vi "Instrument Face Avant.vi"() -> ()   [LabVIEW 2024]
uses:
  <instrlib>/Keithley 2000/Keithley 2000.lvlib
panel:
  in  "Bouton Arrêt du processus":bool
  out "Valeur moyenne":dbl
  out "Valeur max":dbl
  out "Valeur min":dbl
  out "Chaîne":string
  out "Fichier de mesure":path
  out "Graphe":dbl[](graph)
  in  "Nombre de mesures ?":dbl=1.0 min=1.0 step=1.0
  in  "Période (s) ?":dbl=1.0 min=1.0 step=1.0
  in  "Bouton EXECUTER":bool
  in  "Bouton CONFIGURER":bool
  in  "Fonction":u16(ring) items=["TENSION DC", "TENSION AC", "COURANT DC", "COURANT AC", "RESISTANCE 2 points", "RESISTANCE 4 points", "FREQUENCE", "TEMPERATURE"]
  in  "Message d'accueil":string(combo)
  # "MODULE D'ACQUISITION ET DE TRAITEMENT DE DONNEES"
  # "RESULTATS DES MESURES"
  # "CONFIGURATION DE L'INSTRUMENT"
  # "CONFIGURATION DE L'ACQUISITION"
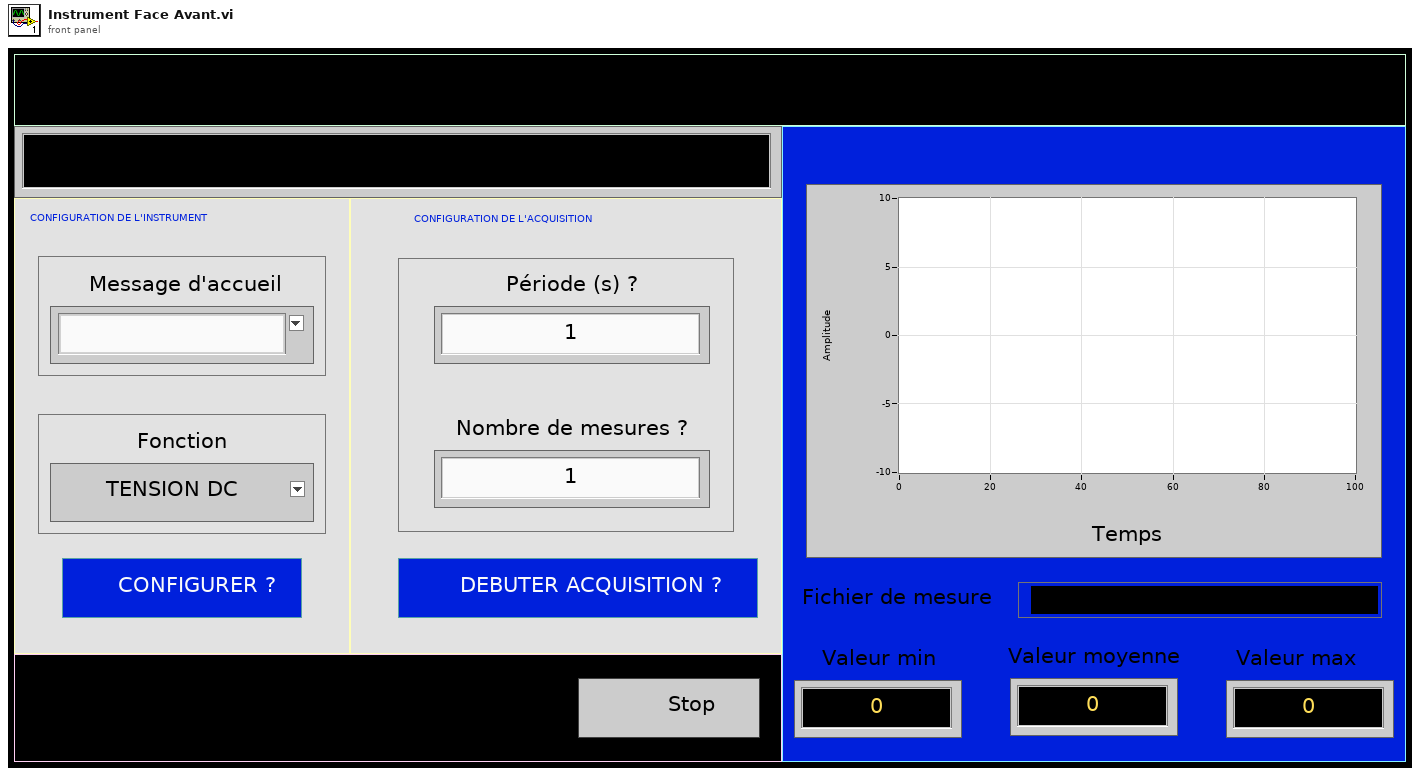
[diagram p1: front panel]
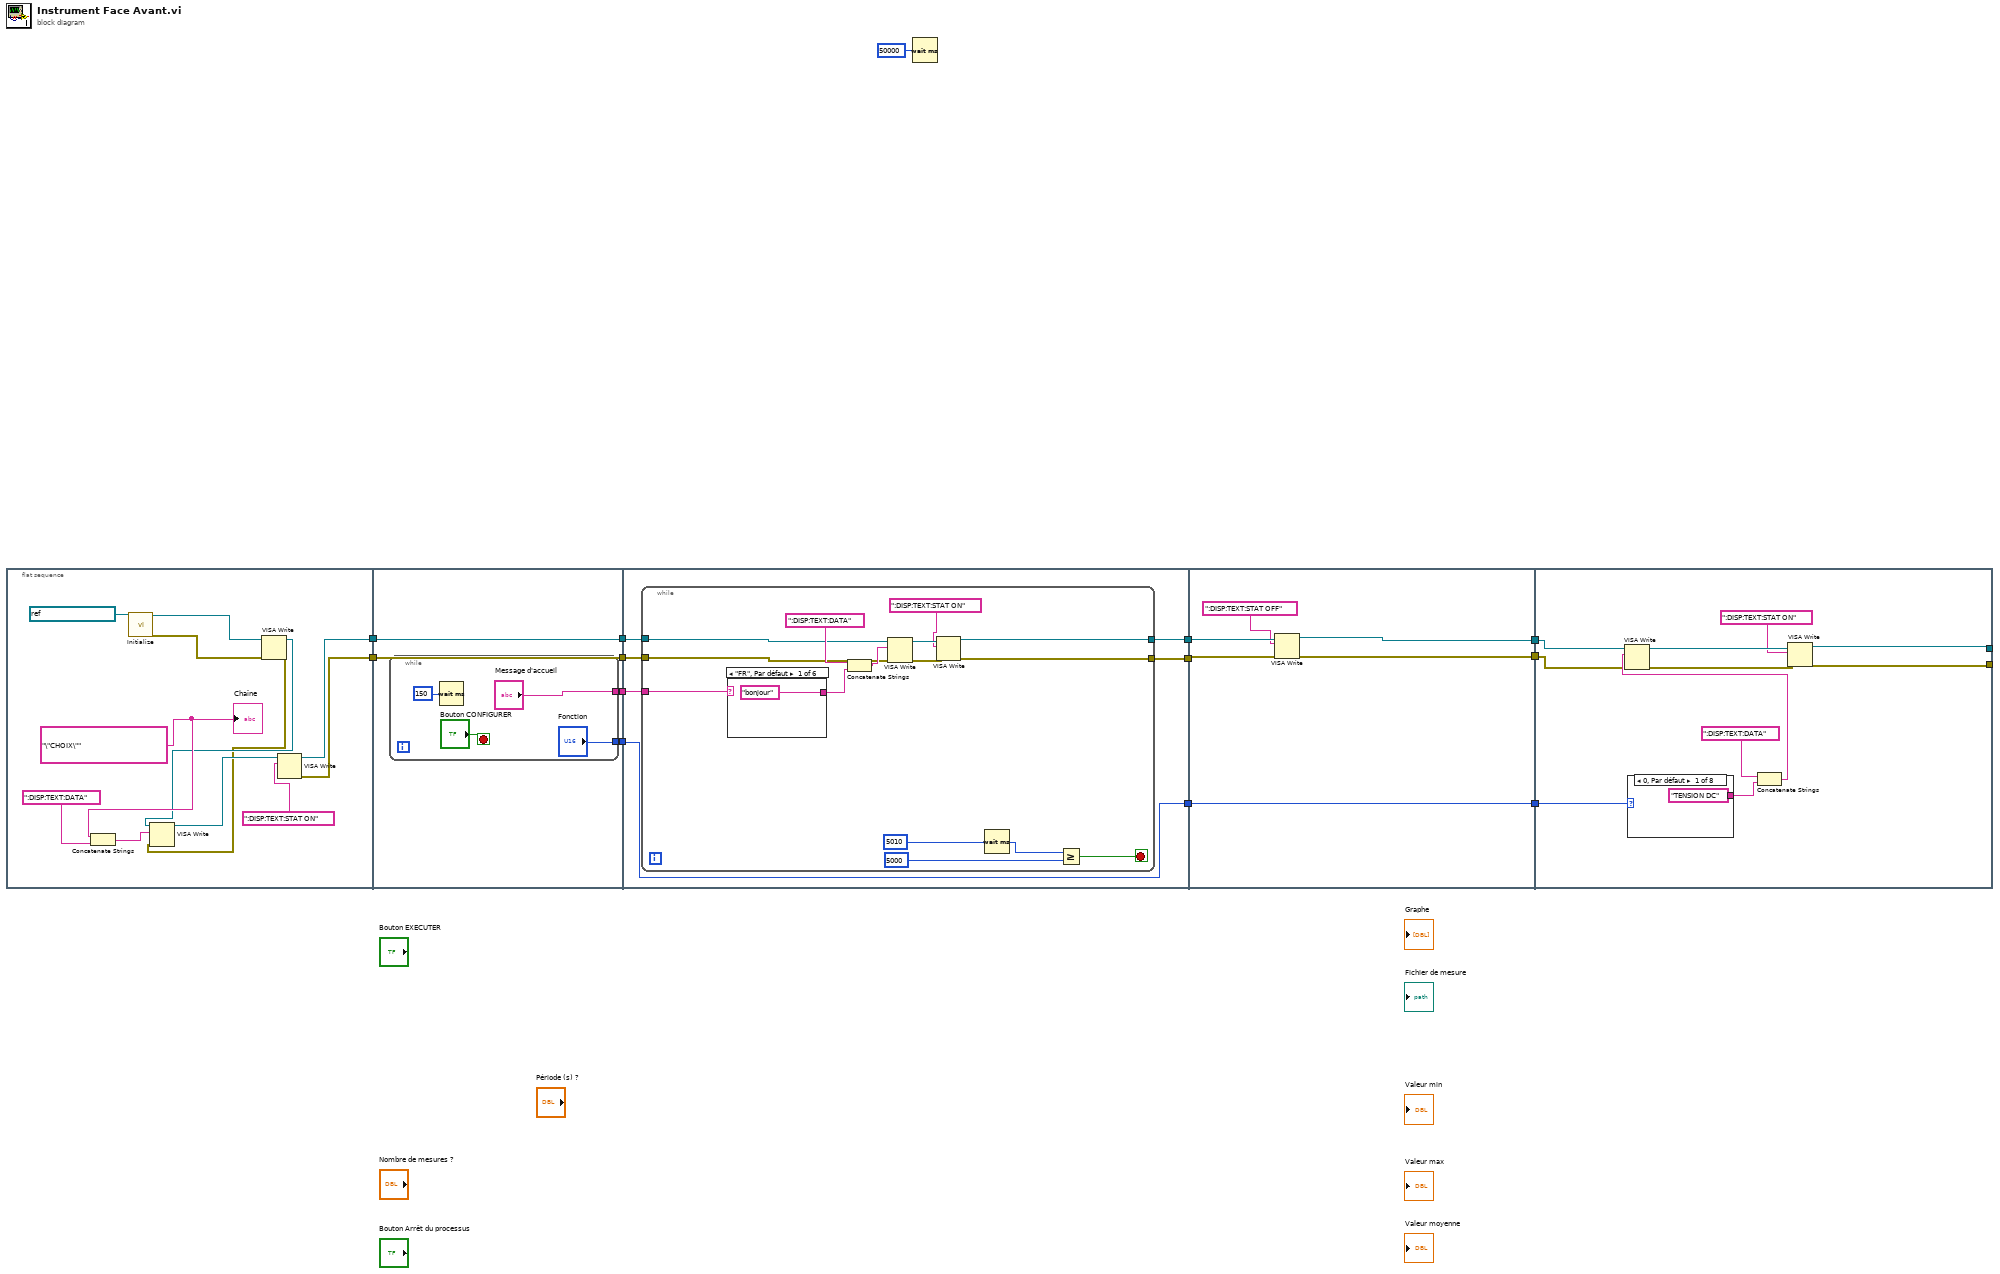
[diagram p0: block diagram]
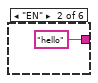
[diagram p2: hidden frame]
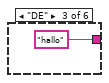
[diagram p3: hidden frame]
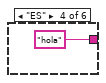
[diagram p4: hidden frame]
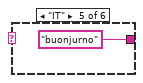
[diagram p5: hidden frame]
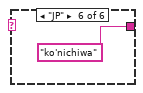
[diagram p6: hidden frame]
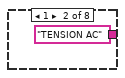
[diagram p7: hidden frame]
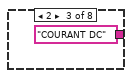
[diagram p8: hidden frame]
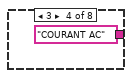
[diagram p9: hidden frame]
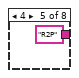
[diagram p10: hidden frame]
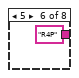
[diagram p11: hidden frame]
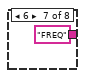
[diagram p12: hidden frame]
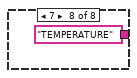
[diagram p13: hidden frame]
diagram:
  n1 = flat-sequence {
    tunnel: [w16] -> w12
    tunnel: [w17] -> w10
    tunnel: [w29] -> w13
    tunnel: w12 -> [w29]
    tunnel: [w28] -> w11
    tunnel: w10 -> [w28]
    tunnel: [w27] -> w5
    tunnel: [w26] -> w2
    tunnel: w13 -> [w39]
    tunnel: w11 -> [w38]
    tunnel: [w37] -> w9
    tunnel: [w36] -> w8
    tunnel: w5 -> [w35]
    tunnel: [w34] -> w3
    tunnel: w2 -> [w34]
    tunnel: w9 -> [w64]
    tunnel: w8 -> [w66]
    tunnel: [w65] -> w7
    tunnel: [w63] -> w6
    tunnel: [w61] -> w4
    tunnel: w3 -> [w61]
    tunnel: w7 -> [w74]
    tunnel: w6 -> [w73]
    tunnel: [w69] -> _
    tunnel: [w68] -> _
    tunnel: w4 -> [w67]
    frame #0 {
      w20 = "\"CHOIX\""
      n2 = Concatenate Strings(w20, ":DISP:TEXT:DATA" ("chaîne")) -> (w22:string)
      n3 = call <instrlib>:"Initialize.vi"("VISA resource name"=refnum<visa-resource-name> "GPIB0::2::INSTR") -> ("VISA resource name out"=w24:refnum<visa-resource-name>, "error out"=w23:errorcluster)  [unwired: 17 in]
      n4 = VISA Write(VISA resource name=w24, error in (no error)=w23) -> (VISA resource name out=w15:refnum<visa-resource-name>, error out=w14:errorcluster)  [unwired: 1 in, 1 out]
      n5 = VISA Write(VISA resource name=w15, write buffer=w22, error in (no error)=w14) -> (VISA resource name out=w19:refnum<visa-resource-name>)  [unwired: 2 out]
      n6 = VISA Write(VISA resource name=w19, write buffer=":DISP:TEXT:STAT ON" ("chaîne")) -> (VISA resource name out=w16:refnum<visa-resource-name>, error out=w17:errorcluster)  [unwired: 1 in, 1 out]
      "Chaîne" <- w20
    }
    frame #1 {
      n7 = while {
        tunnel: ["Message d'accueil"] -> w27
        tunnel: ["Fonction"] -> w26
        stop <- "Bouton CONFIGURER" stop-if-true
        n8 = Wait (ms)(milliseconds to wait=u32 150 ("attente (ms)")) -> ()  [unwired: 1 out]
      }
    }
    frame #2 {
      n9 = while {
        tunnel: w39 -> [w51]
        tunnel: w38 -> [w50]
        tunnel: [w43] -> w37
        tunnel: [w42] -> w36
        tunnel: w35 -> [w40]
        stop <- w44 stop-if-true
        n10 = case shown="\"FR\", Par défaut" w40 {
          tunnel: ["bonjour" "hello" "hallo" "hola" "buonjurno" "ko'nichiwa"] -> w53
          frame "FR", Default {
          }
          frame "EN" {
          }
          frame "DE" {
          }
          frame "ES" {
          }
          frame "IT" {
          }
          frame "JP" {
          }
        }
        n11 = Concatenate Strings(":DISP:TEXT:DATA" ("chaîne"), w53) -> (w54:string)
        n12 = VISA Write(VISA resource name=w51, write buffer=w54, error in (no error)=w50) -> (VISA resource name out=w49:refnum<visa-resource-name>, error out=w48:errorcluster)  [unwired: 1 out]
        n13 = VISA Write(VISA resource name=w49, write buffer=":DISP:TEXT:STAT ON" ("chaîne"), error in (no error)=w48) -> (VISA resource name out=w42:refnum<visa-resource-name>, error out=w43:errorcluster)  [unwired: 1 out]
        n14 = Wait (ms)(milliseconds to wait=u32 5010 ("attente (ms)")) -> (millisecond timer value=w47:u32)
        n15 = Greater Or Equal?(x=w47, y=u32 5000) -> (x >= y?=w44:bool)
      }
    }
    frame #3 {
      n16 = VISA Write(VISA resource name=w66, write buffer=":DISP:TEXT:STAT OFF" ("chaîne"), error in (no error)=w64) -> (VISA resource name out=w65:refnum<visa-resource-name>, error out=w63:errorcluster)  [unwired: 1 out]
    }
    frame #4 {
      n17 = case shown="0, Par défaut" w67 {
        tunnel: ["TENSION DC" "TENSION AC" "COURANT DC" "COURANT AC" "R2P" "R4P" "FREQ" "TEMPERATURE"] -> w77
        frame 0, Default {
        }
        frame 1 {
        }
        frame 2 {
        }
        frame 3 {
        }
        frame 4 {
        }
        frame 5 {
        }
        frame 6 {
        }
        frame 7 {
        }
      }
      n18 = Concatenate Strings(":DISP:TEXT:DATA" ("chaîne"), w77) -> (w75:string)
      n19 = VISA Write(VISA resource name=w74, write buffer=w75, error in (no error)=w73) -> (VISA resource name out=w71:refnum<visa-resource-name>, error out=w72:errorcluster)  [unwired: 1 out]
      n20 = VISA Write(VISA resource name=w71, write buffer=":DISP:TEXT:STAT ON" ("chaîne"), error in (no error)=w72) -> (VISA resource name out=w69:refnum<visa-resource-name>, error out=w68:errorcluster)  [unwired: 1 out]
    }
  }
  n21 = Wait (ms)(milliseconds to wait=u32 50000 ("attente (ms)")) -> ()  [unwired: 1 out]
